vi "ParseHostInfo.vi"(8 "error in":errorcluster, 11 "response":T1) -> (0 "error out":errorcluster, 3 "Cluster":cluster{"IP address":string, "host info":T2})   [LabVIEW 2014, in "Raspberry Pi Compatible Compiler for LabVIEW.lvlib" / "Autodetect.lvlib"]
uses:
  Autodetect.lvlib
  TypeDefs/UDP_HostinfoTD.ctl
  TypeDefs/UDP_Response_TD.ctl
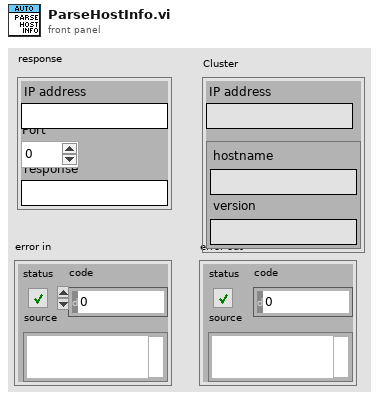
[diagram p1: front panel]
types:
  T1 = typedef "Raspberry Pi Compatible Compiler for LabVIEW.lvlib/Autodetect.lvlib/UDP_Response_TD.ctl" = cluster{"IP address":string, "Port":u16, "response":string}
  T2 = typedef "Raspberry Pi Compatible Compiler for LabVIEW.lvlib/Autodetect.lvlib/UDP_HostinfoTD.ctl" = cluster{"hostname":string, "version":string}
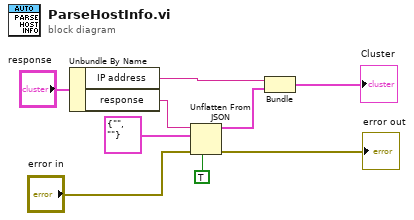
[diagram p0: block diagram]
diagram:
  n1 = Unbundle By Name("response") -> ("IP address"=w8:string, "response"=w1:string)
  n2 = Unflatten From JSON(JSON string=w1, type and defaults=T2 {"hostname"="", "version"=""} ("host info"), default null elements? (F)=TRUE, error in (no error)="error in") -> (value=w3:T2, error out=→"error out":errorcluster)  [unwired: 3 in]
  n3 = Bundle("IP address"=w8, "host info"=w3) -> (→"Cluster":cluster{"IP address":string, "host info":T2})  [unwired: 1 in]
